vi "Get (U16).vi"(8 "error in":errorcluster, 11 "Value in":refnum<class "Value.lvclass">) -> (0 "error out":errorcluster, 1 "Defined?":bool, 2 "Value":u16, 3 "Value out":refnum<class "Value.lvclass">)   [LabVIEW 2019, in "Electronic Datasheet.lvlib" / "Value.lvclass"]
uses:
  Value.lvclass
  Value.lvclass/Value.ctl
  Electronic Datasheet.lvlib
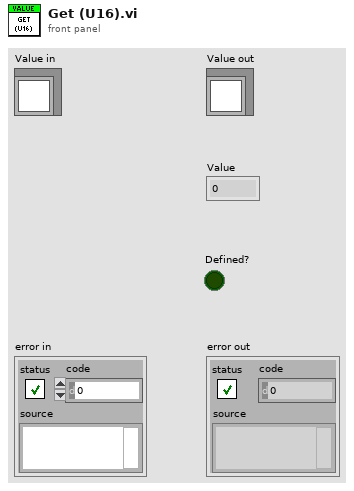
[diagram p1: front panel]
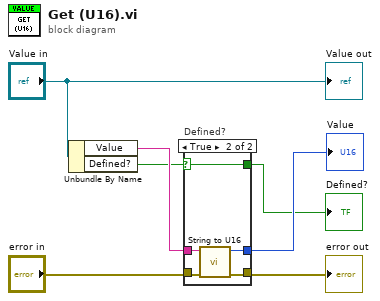
[diagram p0: block diagram]
diagram:
  n1 = Unbundle By Name("Value in") -> ("Value"=w6:string, "Defined?"=w2:bool)
  n2 = case "Defined?" shown="True" w2 {
    selector: w2 -> [w8 w10]
    tunnel: w6 -> [_ w14]
    tunnel: "error in" -> [w9 w13]
    tunnel: [w9 w12] -> w4
    tunnel: [_ w11] -> w3
    tunnel: [w8 w10] -> w1
    frame False {
    }
    frame True {
      n3 = call "String to U16.vi"("error in"=w13, "Integer String"=w14) -> ("error out"=w12:errorcluster, "U16"=w11:u16)  [unwired: 8 in]
    }
  }
  "error out" <- w4
  "Value" <- w3
  "Defined?" <- w1
  "Value out" <- "Value in"
